vi "Pre Launch Init.vi"(11 "Storage Line in":refnum<class "Storage Line.lvclass">) -> (0 "error out":errorcluster, 3 "Storage Line out":refnum<class "Storage Line.lvclass">)   [LabVIEW 2015, in "cRIO-Carbondioxide.lvlib" / "CO2-Actor.lvlib" / "Storage Line.lvclass"]
doc: "(<B>Filename</B>: Actor Framework.lvlib:Actor.lvclass:Pre Launch Init.vi)\n\nDefines behavior that occurs after the Launch Actor method is invoked but before the actor's Actor Core method begins running.\n\nThe Pre Launch Init method is guaranteed to finish before the Launch Actor method returns to its caller and before the actor itself receives any messages. Any references that the Pre Launch Init method obtains are guaranteed to have the same lifetime as the actor itself. Any errors that the Pre Launch Init method returns will abort the launch.\n\nBy default, this method does nothing. A descendant class may override it to define behavior."
uses:
  Storage Line.lvclass
  CO2 Actor Messages/Timeout Msg/Timeout Msg.lvclass
  <vilib>/ActorFramework/Message Enqueuer/Message Priority.ctl
  Storage Line.lvclass/Storage Line.ctl
  <vilib>/ActorFramework/Actor/Actor.lvclass/Actor.ctl
  <vilib>/ActorFramework/Message Enqueuer/Message Enqueuer.lvclass/Message Enqueuer.ctl
  Storage Line Messages/Set Line Msg/Set Line Msg.lvclass/Set Line Msg.ctl
  <vilib>/ActorFramework/Actor/Read Self Enqueuer.vi
  <vilib>/ActorFramework/Message Enqueuer/Enqueue.vi
  <vilib>/ActorFramework/Message Enqueuer/Init from Existing Queue.vi
  <vilib>/ActorFramework/Message Priority Queue/Priority Enqueue.vi
  CO2 Actor/CO2 Actor.lvclass
  Storage Line Messages/Set Line Msg/Set Line Msg.lvclass
  Interlocks/Interlock Chain/Interlock Chain.lvclass
  Storage Line Messages/Launch Valves Msg/Launch Valves Msg 2.lvclass
  <vilib>/ActorFramework/Message Enqueuer/Message Enqueuer.lvclass
  <vilib>/ActorFramework/Actor/Actor.lvclass
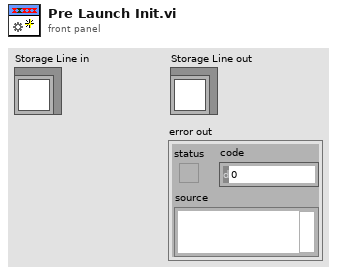
[diagram p1: front panel]
types:
  T1 = typedef "Actor Framework.lvlib/Message Enqueuer.lvclass/Message Priority.ctl" = enum16{"Low", "Normal", "High"}
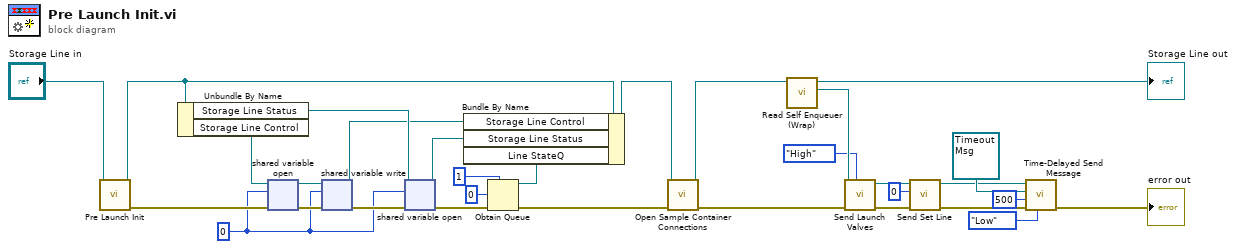
[diagram p0: block diagram]
diagram:
  w25 = u16 0
  n1 = call-parent "Pre Launch Init.vi"("CO2 Actor in"="Storage Line in") -> ("error out"=w27:errorcluster, "CO2 Actor out"=w24:refnum<class "Storage Line.lvclass">)  [unwired: 9 in]
  n2 = Unbundle By Name(w24) -> ("Storage Line Status"=w23:refnum<k21>, "Storage Line Control"=w26:refnum<k21>)
  n3 = shared-variable-open(w26, w27, w25) -> (w28:refnum<k21>, w30:errorcluster)  [unwired: 1 in]
  n4 = shared-variable-write(w28, w30, w25) -> (w22:refnum<k21>, w29:errorcluster)
  n5 = shared-variable-open(w23, w29, w25) -> (w21:refnum<k21>, w5:errorcluster)  [unwired: 1 in]
  n6 = Obtain Queue(max queue size (-1, unlimited)=1, element data type=u16 0, error in (no error)=w5) -> (queue out=w1:refnum<queue>, error out=w4:errorcluster)  [unwired: 2 in, 1 out]
  n7 = Bundle By Name(cluster=w24, "Storage Line Control"=w22, "Storage Line Status"=w21, "Line StateQ"=w1) -> (w10:refnum<class "Storage Line.lvclass">)
  n8 = call "Open Sample Container Connections.vi"("error in (no error)"=w4, "Storage Line in"=w10) -> ("error out"=w8:errorcluster, "Storage Line out"=w9:refnum<class "Storage Line.lvclass">)  [unwired: 8 in]
  n9 = call "Read Self Enqueuer (Wrap).vi"("CO2 Actor in"=w9) -> ("Actor Framework:Message Enqueuer"=w17:refnum<class "Message Enqueuer.lvclass">, "CO2 Actor out"=→"Storage Line out":refnum<class "Storage Line.lvclass">)  [unwired: 9 in]
  n10 = call "Send Launch Valves.vi"("Message Priority (Normal)"=Message_Priority."High", "error in (no error)"=w8, "Message Enqueuer"=w17) -> ("error out"=w13:errorcluster, "Message Enqueuer out"=w15:refnum<class "Message Enqueuer.lvclass">)  [unwired: 7 in]
  n11 = call "Send Set Line.vi"("error in (no error)"=w13, "Bit Field"=u16 0, "Message Enqueuer"=w15) -> ("error out"=w12:errorcluster, "Message Enqueuer out"=w14:refnum<class "Message Enqueuer.lvclass">)  [unwired: 7 in]
  n12 = call <vilib>:"Time-Delayed Send Message.vi"("Message Priority (Normal)"=Message_Priority."Low", "error in (no error)"=w12, "Milliseconds To Wait"=500, "Message"=refnum<class "Timeout Msg.lvclass"> refnum ("Timeout Msg.lvclass"), "Message Enqueuer"=w14) -> ("error out"=→"error out":errorcluster)  [unwired: 5 in, 1 out]
